vi "get_hostMessages.vi"(0 "Host_Reference":refnum<class "HGF_Reference.lvclass">, 2 "timeout in ms (-1)":i32=-1, 5 "error in (no error)":errorcluster) -> (14 "dup Host_Reference":refnum<class "HGF_Reference.lvclass">, 16 "Host Messages":refnum<class "MoAgSy_Message.lvclass">[](array[class]), 17 "Message(s)?":bool, 19 "error out":errorcluster)   [LabVIEW 2009, in "MoAgSy.lvlib" / "MoAgSy_Host.lvclass"]
doc: "<B>public</B> VI returns referenced Hosts messages.\nNew messages are submitted internally using a queue.\n\nF.Berck@gsi.de\nGSI Darmstadt 2009"
uses:
  MoAgSy_Host.lvclass
  HGF_BaseClasses/HGF_Reference/HGF_Reference.lvclass
  MoAgSy_Message/MoAgSy_Message.lvclass
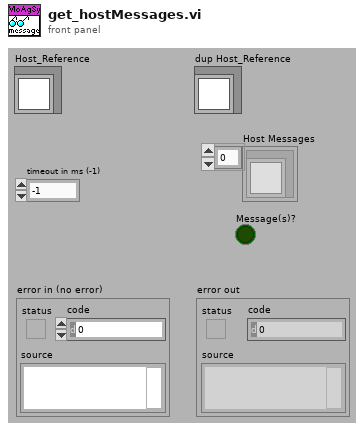
[diagram p1: front panel]
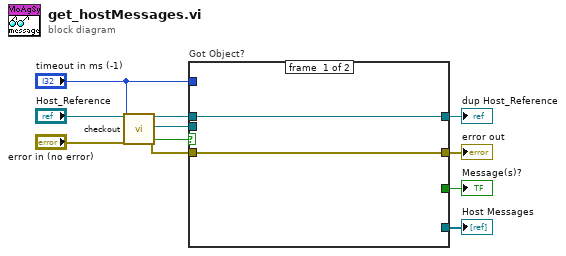
[diagram p0: block diagram]
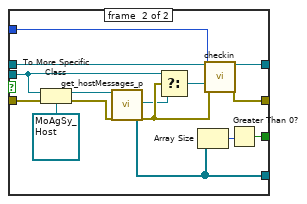
[diagram p2: hidden frame]
diagram:
  n1 = call "checkout.vi"("HGF_Reference"="Host_Reference", "timeout in ms (-1)"="timeout in ms (-1)", "error in (no error)"="error in (no error)") -> ("dup HGF_Reference"=w6:refnum<class "HGF_Reference.lvclass">, "Object"=w4:refnum<class>, "got object?"=w5:bool, "error out"=w3:errorcluster)  [unwired: 13 out]
  n2 = case "Got Object?" shown="True" w5 {
    tunnel: w4 -> [_ w20]
    tunnel: w6 -> [w13 w26]
    tunnel: [w13 w25] -> w10
    tunnel: "timeout in ms (-1)" -> [_ w24]
    tunnel: [w12 w23] -> w9
    tunnel: w3 -> [w12 w22]
    tunnel: [_ w16] -> w2
    tunnel: [_ w14] -> w1
    frame #0 {
    }
    frame #1 {
      n3 = To More Specific Class(target class=refnum<class "MoAgSy_Host.lvclass"> refnum ("MoAgSy.lvlib:MoAgSy_Host.lvclass"), reference=w20, error in=w22) -> (specific class reference=w19:refnum<class "MoAgSy_Host.lvclass">, error out=w17:errorcluster)
      n4 = call "get_hostMessages_p.vi"("MoAgSy_Host"=w19, "error in (no error)"=w17) -> ("dup MoAgSy_Host"=w18:refnum<class "MoAgSy_Host.lvclass">, "Host Messages"=w16:refnum<class "MoAgSy_Message.lvclass">[], "error out"=w28:errorcluster)  [unwired: 15 out]
      n5 = Select(t=w20, s=w28, f=w18) -> (s? t:f=w21:refnum<class>)
      n6 = Array Size(array=w16) -> (size(s)=w15:i32)
      n7 = call "checkin.vi"("HGF_Reference"=w26, "Object"=w21, "timeout /ms (-1)"=w24, "error in (no error)"=w28) -> ("dup HGF_Reference"=w25:refnum<class "HGF_Reference.lvclass">, "error out"=w23:errorcluster)  [unwired: 14 out]
      n8 = Greater Than 0?(x=w15) -> (x > 0?=w14:bool)
    }
  }
  "dup Host_Reference" <- w10
  "error out" <- w9
  "Host Messages" <- w2
  "Message(s)?" <- w1
